vi "display_michelle_PTK_visjitter_stopadded_RandCont_PsuedoCO_TSLog.vi"() -> ()   [LabVIEW 2019]
uses:
  <vilib>/Analysis/Matrix/Datatypes/RealMatrix.ctl
  <vilib>/Utility/file.llb/Write Delimited Spreadsheet (DBL).vi
  <vilib>/Analysis/Matrix/NI_Matrix.lvlib
panel:
  out "lambda":dbl
  out "maxITI":dbl
  out "minITI":dbl
  out "goEXP":dbl
  out "meanITI":dbl
  out "Lag1":dbl
  out "TSLog":dbl[][](array[numeric])
  out "TSLog2":dbl[][](array[numeric])
  out "Initialtime":dbl
  out "Time Stamp":timestamp format="%<%H:%M:%S%4u>T"
  out "TSLog1":dbl[][](array[numeric])
  out "ArrayTemp3":T1
  out "StimID2":dbl
  out "Contrast":dbl
  out "TimeOutCounter":i32
  out "ElapsedTime_M":dbl
  out "Base_Contrast":dbl
  out "CurrentTrial":u32=1
  out "Jitter":dbl
  out "BaseITI":dbl
  out "VisStimDuration":dbl
  in  "Stop":bool
  out "Num trials":u32=204
  out "ISI Time":dbl
  out "Stim TS":dbl
  out "Output":dbl[][](array[numeric])
  out "Output frame":T1
  out "Array temp1":T1
  out "Elapsed Time":dbl
  out "Display":bool=TRUE
  out "Trial":u32=1
  out "reward":dbl[](array[numeric])
  out "stim_id":dbl[](array[numeric])
  out "stim_loaded":dbl
  out "Timings":dbl[](array[numeric])
  out "Stimuli Loaded?":bool
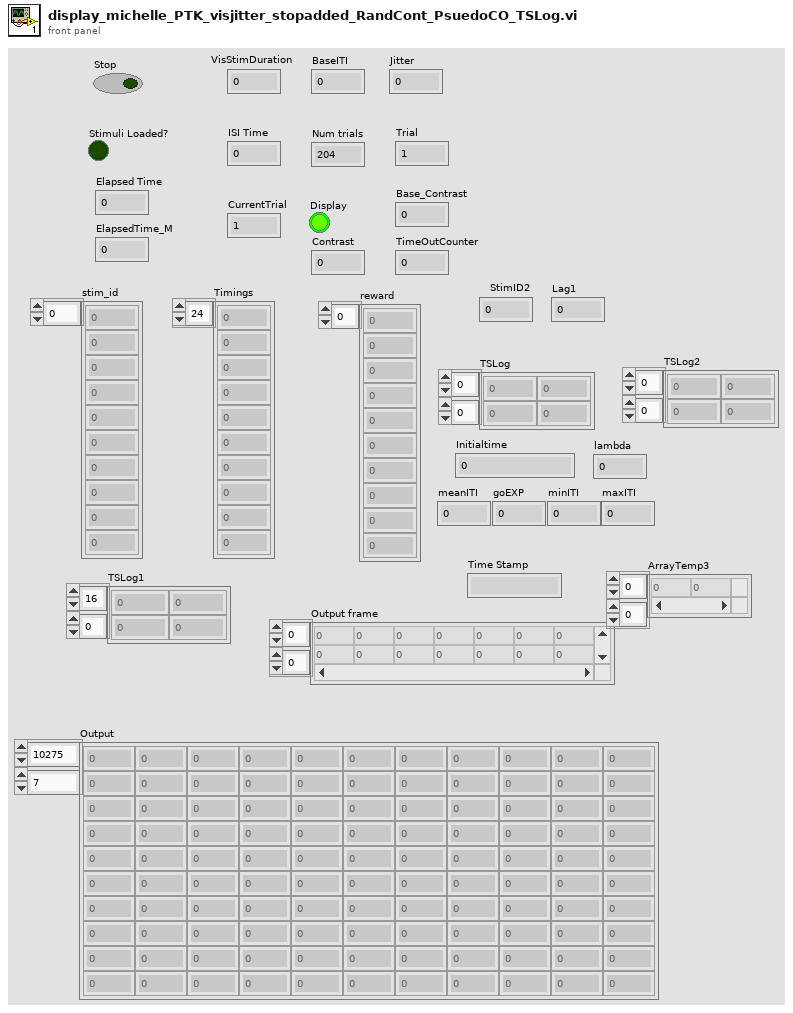
[diagram p1: front panel]
types:
  T1 = typedef "NI_Matrix.lvlib/RealMatrix.ctl" = dbl[][]
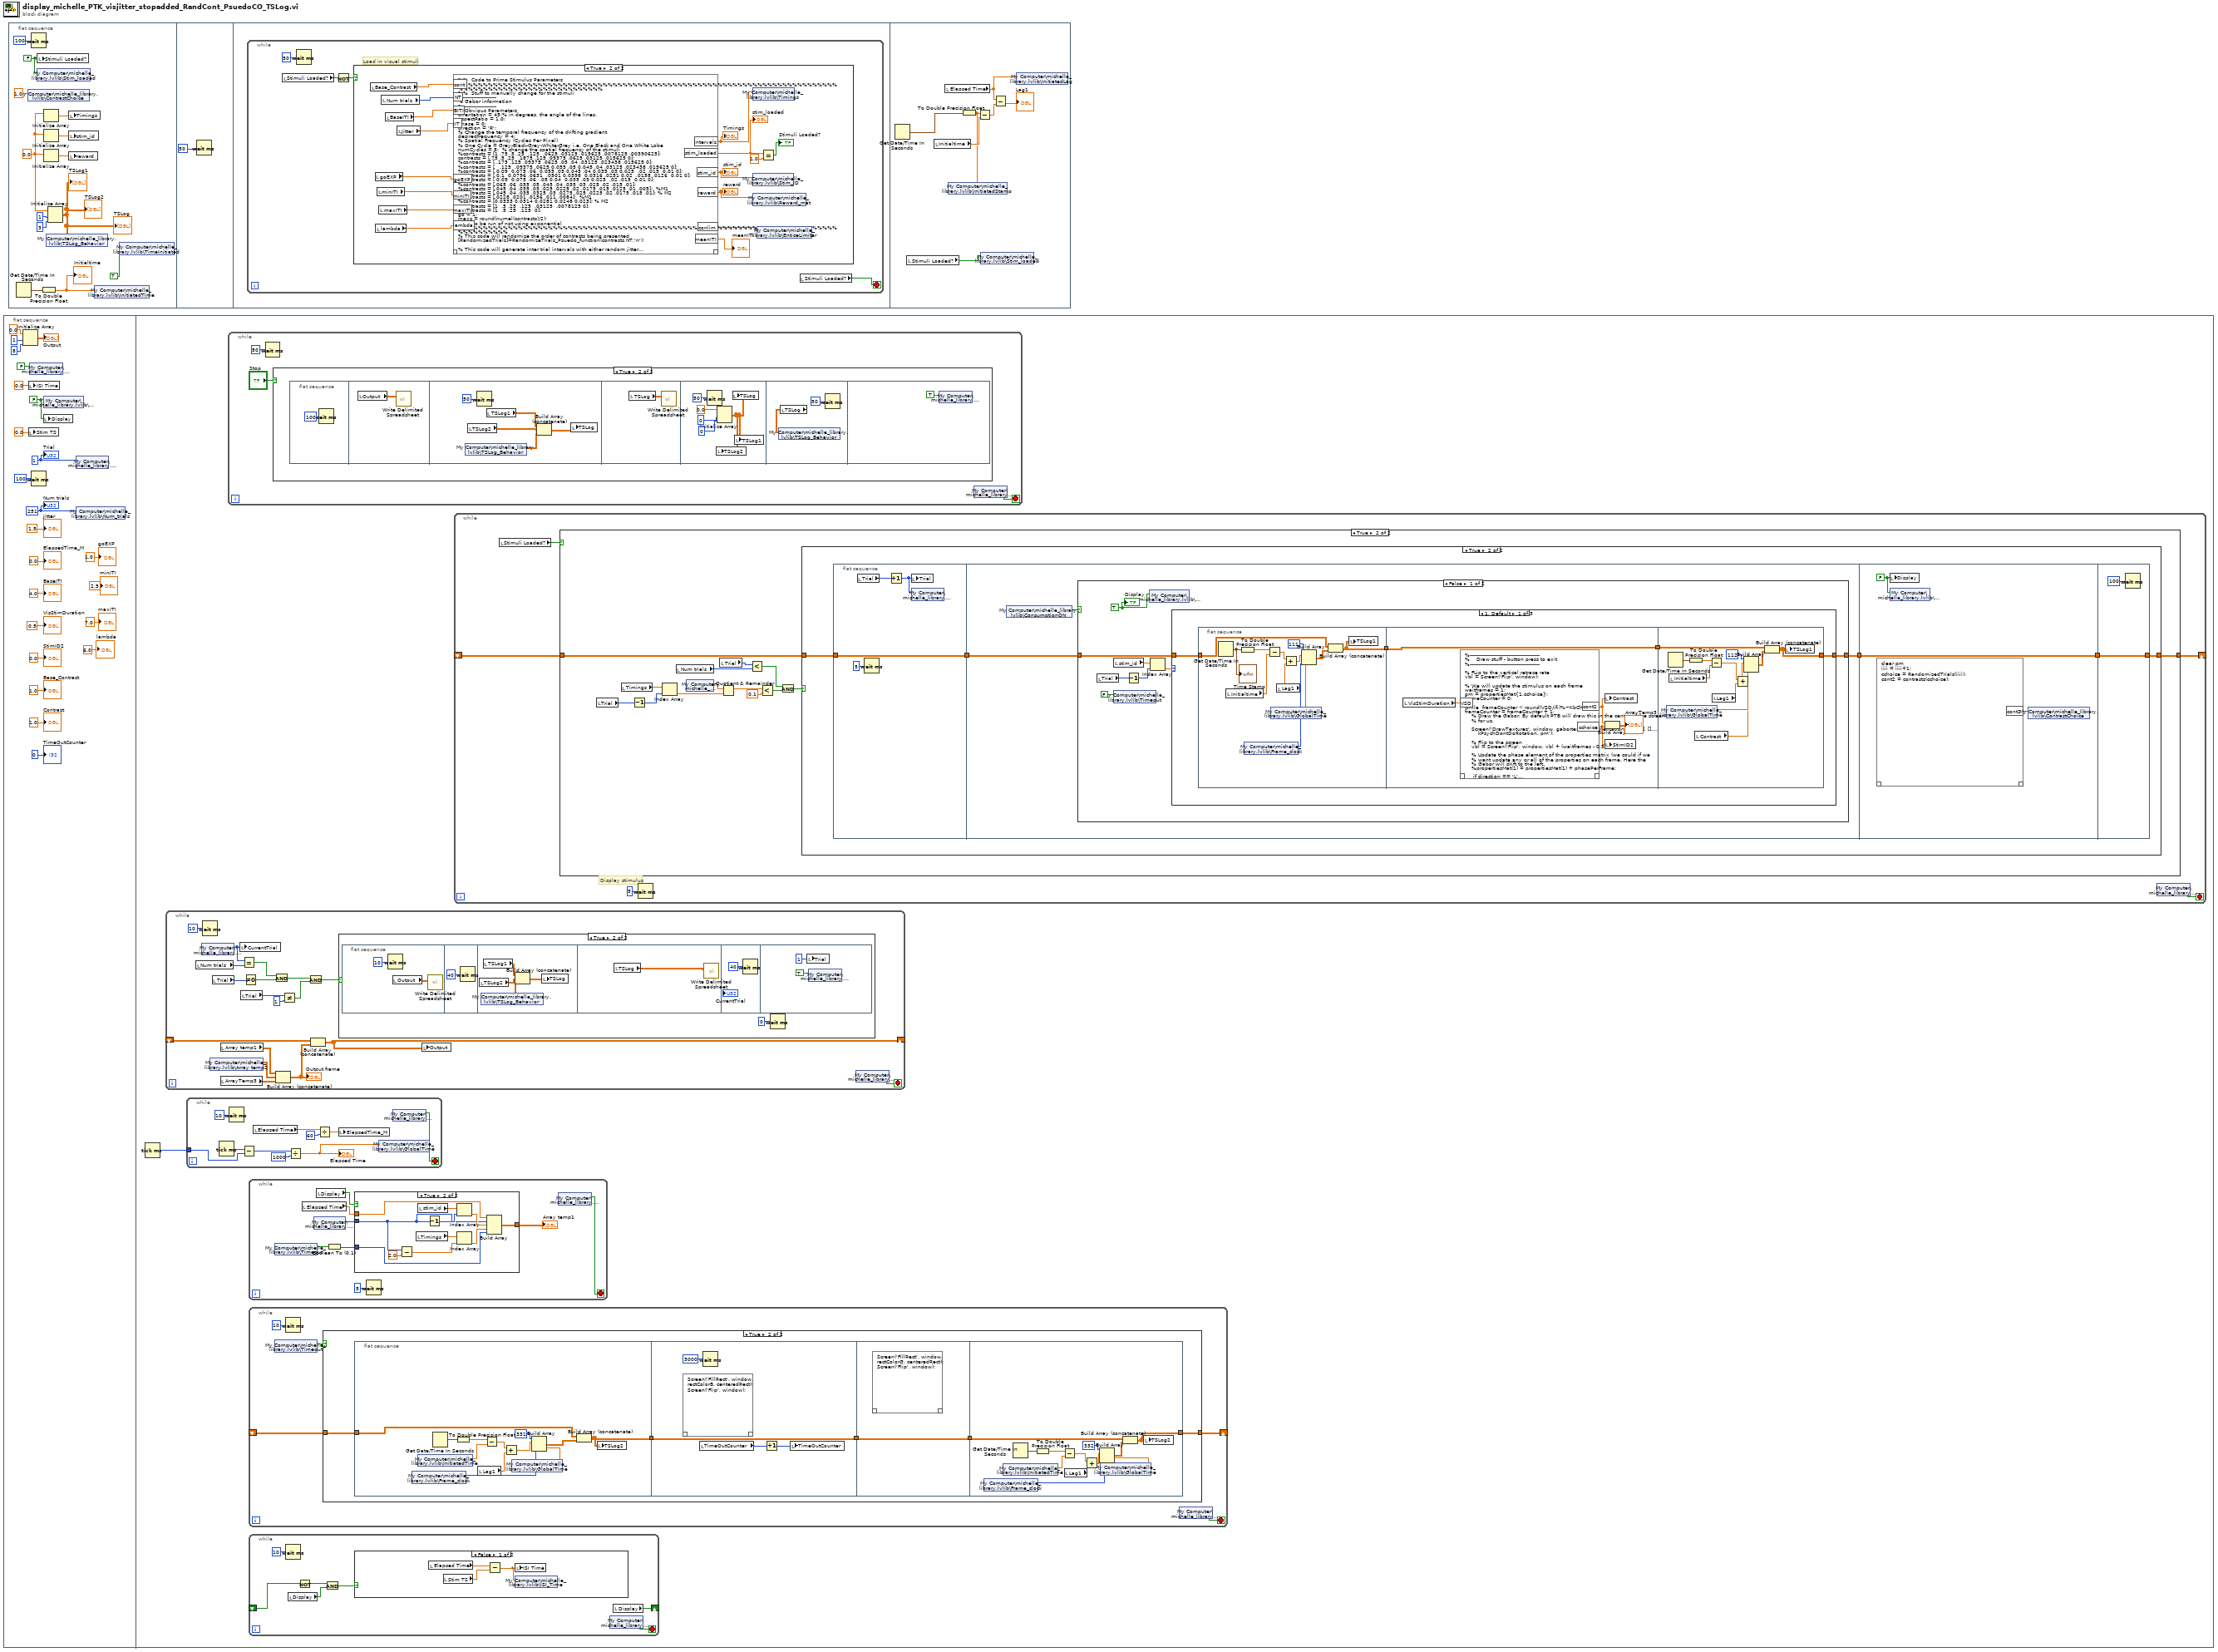
[diagram p0: block diagram]
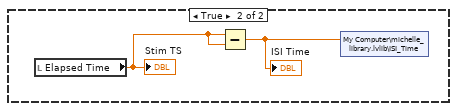
[diagram p5: hidden frame]
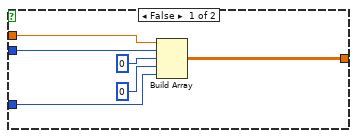
[diagram p6: hidden frame]
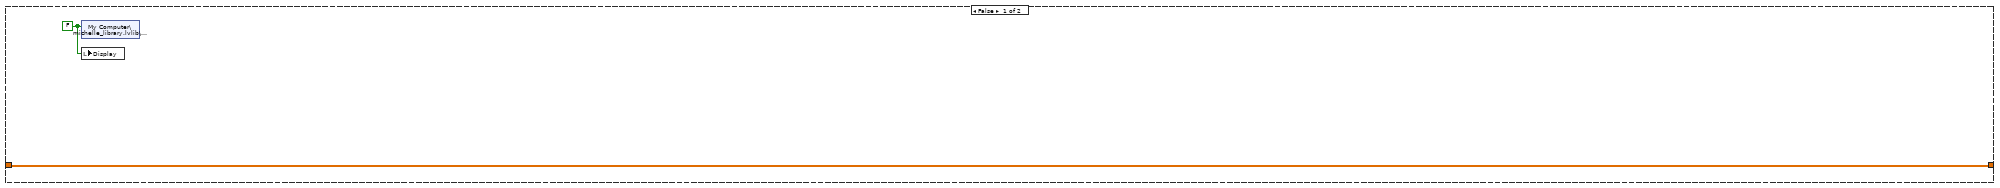
[diagram p9: hidden frame]
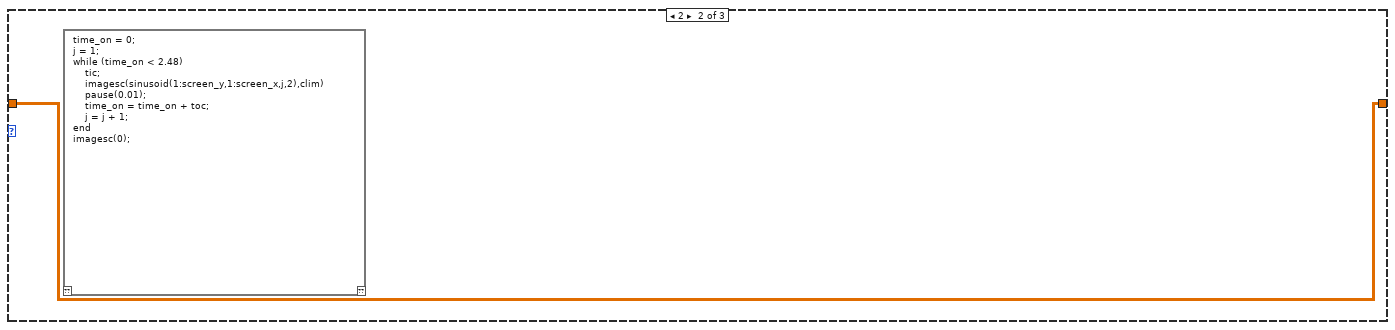
[diagram p10: hidden frame]
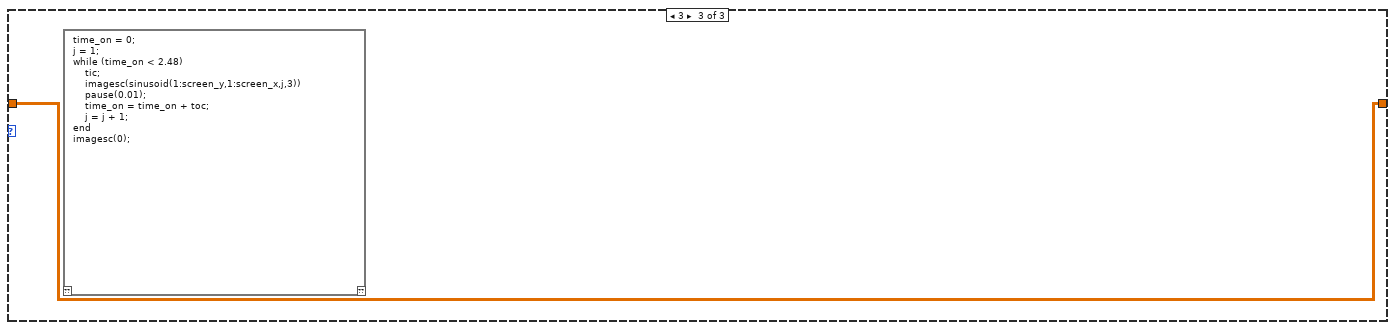
[diagram p11: hidden frame]
diagram:
  n1 = flat-sequence {
    frame #0 {
      w15 = u32 251
      w21 = FALSE ("Display")
      w23 = u32 1 ("Trial")
      n2 = Initialize Array(0.0 ("element"), 1 ("dimension size"), 8 ("dimension size")) -> (→"Output":dbl[][])
      n3 = local write "ISI Time"(0.0 ("ISI Time")) -> ()
      n4 = local write "Stim TS"(0.0 ("Stim TS")) -> ()
      n5 = shared-variable "My Computer\\michelle_library.lvlib\\Stop"(FALSE ("Stop")) -> ()  [unwired: 1 in, 1 out]
      n6 = Wait (ms)(milliseconds to wait=u32 100) -> ()  [unwired: 1 out]
      n7 = shared-variable "My Computer\\michelle_library.lvlib\\Display"(w21) -> ()  [unwired: 1 in, 1 out]
      n8 = local write "Display"(w21) -> ()
      n9 = shared-variable "My Computer\\michelle_library.lvlib\\Trial"(w23) -> ()  [unwired: 1 in, 1 out]
      n10 = shared-variable "My Computer\\michelle_library.lvlib\\Num_trials"(w15) -> ()  [unwired: 1 in, 1 out]
      "Trial" <- w23
      "Num trials" <- w15
      "VisStimDuration" <- 0.5
      "BaseITI" <- 4.0
      "Jitter" <- 1.5
      "Base_Contrast" <- 1.0
      "ElapsedTime_M" <- 0.0
      "TimeOutCounter" <- 0
      "Contrast" <- 1.0
      "StimID2" <- 0.0
      "goEXP" <- 1.0
      "minITI" <- 2.5
      "maxITI" <- 7.0
      "lambda" <- 6.0
    }
    frame #1 {
      n11 = Tick Count (ms)() -> (millisecond timer value=w24:u32)
      n12 = while {
        shift-right: [w145] -> _
        shift-left: _ -> [w146]
        stop <- w148 stop-if-true
        n13 = local read "Num trials"() -> (w141:u32)
        n14 = shared-variable "My Computer\\michelle_library.lvlib\\Trial"() -> (w132:u32)  [unwired: 1 in, 1 out]
        n15 = Wait (ms)(milliseconds to wait=u32 10) -> ()  [unwired: 1 out]
        n16 = shared-variable "My Computer\\michelle_library.lvlib\\Array temp2"() -> (w143:dbl[][])  [unwired: 1 in, 1 out]
        n17 = local read "Trial"() -> (w139:u32)
        n18 = local read "Array temp1"() -> (w144:T1)
        n19 = local read "ArrayTemp3"() -> (w131:T1)
        n20 = local write "CurrentTrial"(w132) -> ()
        n21 = local read "Trial"() -> (w138:u32)
        n22 = Equal?(x=w132, y=w141) -> (x = y?=w140:bool)
        n23 = Not Equal To 0?(x=w139) -> (x != 0?=w135:bool)
        n24 = And(x=w140, y=w135) -> (x .and. y?=w133:bool)
        n25 = Build Array (concatenate)(w144, w143, w131) -> (w142:T1)
        "Output frame" <- w142
        n26 = Not Equal?(x=w138, y=1) -> (x != y?=w137:bool)
        n27 = And(x=w133, y=w137) -> (x .and. y?=w134:bool)
        n28 = Build Array (concatenate) ("Build Matrix")(w146, w142) -> (w145:T1)
        n29 = case shown="True" w134 {
          frame False {
          }
          frame True {
            n30 = flat-sequence {
              frame #0 {
                n31 = Wait (ms)(milliseconds to wait=u32 10) -> ()  [unwired: 1 out]
                n32 = local read "Output"() -> (w151:dbl[][])
                n33 = call-poly <vilib>:"Write Delimited Spreadsheet.vi"("2D data"=w151) -> ()  [unwired: 13 in, 2 out]
              }
              frame #1 {
                n34 = Wait (ms)(milliseconds to wait=u32 40) -> ()  [unwired: 1 out]
              }
              frame #2 {
                n35 = local read "TSLog2"() -> (w156:dbl[][])
                n36 = shared-variable "My Computer\\michelle_library.lvlib\\TSLog_Behavior"() -> (w154:dbl[][])  [unwired: 1 in, 1 out]
                n37 = local read "TSLog1"() -> (w155:dbl[][])
                n38 = Build Array (concatenate) ("Build Matrix")(w155, w156, w154) -> (w153:T1)
                n39 = local write "TSLog"(w153) -> ()
              }
              frame #3 {
                n40 = local read "TSLog"() -> (w157:dbl[][])
                n41 = call-poly <vilib>:"Write Delimited Spreadsheet.vi"("2D data"=w157) -> ()  [unwired: 13 in, 2 out]
              }
              frame #4 {
                n42 = Wait (ms)(milliseconds to wait=u32 40) -> ()  [unwired: 1 out]
              }
              frame #5 {
                n43 = local write "Trial"(1) -> ()
                n44 = shared-variable "My Computer\\michelle_library.lvlib\\Stop"(TRUE) -> ()  [unwired: 1 in, 1 out]
              }
            }
            n45 = Wait (ms)(milliseconds to wait=0) -> ()  [unwired: 1 out]
          }
        }
        n46 = local write "Output"(w145) -> ()
        n47 = shared-variable "My Computer\\michelle_library.lvlib\\Stop"() -> (w148:bool)  [unwired: 1 in, 1 out]
      }
      n48 = while {
        tunnel: w24 -> [w128]
        stop <- w125 stop-if-true
        n49 = Tick Count (ms)() -> (millisecond timer value=w129:u32)
        n50 = Wait (ms)(milliseconds to wait=u32 10) -> ()  [unwired: 1 out]
        n51 = Subtract(x=w129, y=w128) -> (x-y=w126:u32)
        n52 = local read "Elapsed Time"() -> (w123:dbl)
        n53 = Divide(x=w126, y=u32 1000) -> (x/y=w121:dbl)
        "Elapsed Time" <- w121
        n54 = Divide(x=w123, y=60) -> (x/y=w122:dbl)
        n55 = local write "ElapsedTime_M"(w122) -> ()
        n56 = shared-variable "My Computer\\michelle_library.lvlib\\GlobalTime"(w121) -> ()  [unwired: 1 in, 1 out]
        n57 = shared-variable "My Computer\\michelle_library.lvlib\\Stop"() -> (w125:bool)  [unwired: 1 in, 1 out]
      }
      n58 = while {
        stop <- w27 stop-if-true
        n59 = Wait (ms)(milliseconds to wait=50) -> ()  [unwired: 1 out]
        n60 = case shown="True" "Stop" {
          frame False {
          }
          frame True {
            n61 = flat-sequence {
              frame #0 {
                n62 = Wait (ms)(milliseconds to wait=100) -> ()  [unwired: 1 out]
              }
              frame #1 {
                n63 = local read "Output"() -> (w29:dbl[][])
                n64 = call-poly <vilib>:"Write Delimited Spreadsheet.vi"("2D data"=w29) -> ()  [unwired: 13 in, 2 out]
              }
              frame #2 {
                n65 = shared-variable "My Computer\\michelle_library.lvlib\\TSLog_Behavior"() -> (w30:dbl[][])  [unwired: 1 in, 1 out]
                n66 = local read "TSLog2"() -> (w33:dbl[][])
                n67 = Wait (ms)(milliseconds to wait=50) -> ()  [unwired: 1 out]
                n68 = local read "TSLog1"() -> (w32:dbl[][])
                n69 = Build Array (concatenate) ("Build Matrix")(w32, w33, w30) -> (w31:T1)
                n70 = local write "TSLog"(w31) -> ()
              }
              frame #3 {
                n71 = local read "TSLog"() -> (w35:dbl[][])
                n72 = call-poly <vilib>:"Write Delimited Spreadsheet.vi"("2D data"=w35) -> ()  [unwired: 13 in, 2 out]
              }
              frame #4 {
                n73 = Wait (ms)(milliseconds to wait=50) -> ()  [unwired: 1 out]
                n74 = Initialize Array(0.0, 0, 0) -> (w37:dbl[][])
                n75 = local write "TSLog2"(w37) -> ()
                n76 = local write "TSLog"(w37) -> ()
                n77 = local write "TSLog1"(w37) -> ()
              }
              frame #5 {
                n78 = local read "TSLog"() -> (w42:dbl[][])
                n79 = shared-variable "My Computer\\michelle_library.lvlib\\TSLog_Behavior"(w42) -> ()  [unwired: 1 in, 1 out]
                n80 = Wait (ms)(milliseconds to wait=50) -> ()  [unwired: 1 out]
              }
              frame #6 {
                n81 = shared-variable "My Computer\\michelle_library.lvlib\\Stop"(TRUE) -> ()  [unwired: 1 in, 1 out]
              }
            }
          }
        }
        n82 = shared-variable "My Computer\\michelle_library.lvlib\\Stop"() -> (w27:bool)  [unwired: 1 in, 1 out]
      }
      n83 = while {
        stop <- w98 stop-if-true
        n84 = shared-variable "My Computer\\michelle_library.lvlib\\Timeout"() -> (w96:bool)  [unwired: 1 in, 1 out]
        n85 = local read "Elapsed Time"() -> (w102:dbl)
        n86 = shared-variable "My Computer\\michelle_library.lvlib\\Trial"() -> (w100:u32)  [unwired: 1 in, 1 out]
        n87 = local read "Display"() -> (w99:bool)
        n88 = Boolean To (0,1)(Boolean=w96) -> (0, 1=w97:i16)
        n89 = case shown="True" w99 {
          tunnel: w100 -> [w108 w111]
          tunnel: w102 -> [w109 w118]
          tunnel: [w107 w119] -> w101
          tunnel: w97 -> [w104 w113]
          frame False {
            n90 = Build Array(w109, w108, u32 0 ("milliseconds to wait"), 0, w104) -> (w107:T1)
          }
          frame True {
            n91 = Subtract(x=w111, y=2.0) -> (x-y=w110:dbl)
            n92 = local read "Timings"() -> (w116:dbl[])
            n93 = local read "stim_id"() -> (w120:dbl[])
            n94 = Decrement(x=w111) -> (x-1=w115:u32)
            n95 = Index Array(array=w120, index=w115) -> (element=w117:dbl)
            n96 = Index Array(array=w116, index=w110) -> (element=w114:dbl)
            n97 = Build Array(w118, w111, w117, w114, w113) -> (w119:T1)
          }
        }
        "Array temp1" <- w101
        n98 = Wait (ms)(milliseconds to wait=u32 5) -> ()  [unwired: 1 out]
        n99 = shared-variable "My Computer\\michelle_library.lvlib\\Stop"() -> (w98:bool)  [unwired: 1 in, 1 out]
      }
      n100 = while {
        shift-right: [w44] -> _
        shift-left: _ -> [w45]
        stop <- w48 stop-if-true
        n101 = shared-variable "My Computer\\michelle_library.lvlib\\Timeout"() -> (w46:bool)  [unwired: 1 in, 1 out]
        n102 = Wait (ms)(milliseconds to wait=u32 10) -> ()  [unwired: 1 out]
        n103 = case shown="True" w46 {
          tunnel: w45 -> [w49 w54]
          tunnel: [w49 w53] -> w44
          frame False {
          }
          frame True {
            n104 = flat-sequence {
              tunnel: w54 -> [w61]
              tunnel: [w60] -> w51
              tunnel: [w67] -> w52
              tunnel: w51 -> [w67]
              tunnel: w52 -> [w71]
              tunnel: [w71] -> w50
              tunnel: [w77] -> w53
              tunnel: w50 -> [w78]
              frame #0 {
                n105 = shared-variable "My Computer\\michelle_library.lvlib\\Frame_clock"() -> (w55:u32)  [unwired: 1 in, 1 out]
                n106 = shared-variable "My Computer\\michelle_library.lvlib\\InitiatedTime"() -> (w64:dbl)  [unwired: 1 in, 1 out]
                n107 = Get Date/Time In Seconds() -> (seconds since 1Jan1904=w66:timestamp)
                n108 = To Double Precision Float(number=w66) -> (double precision float=w65:dbl)
                n109 = local read "Lag1"() -> (w57:dbl)
                n110 = Subtract(x=w65, y=w64) -> (x-y=w58:dbl)
                n111 = Add(x=w58, y=w57) -> (x+y=w59:dbl)
                n112 = shared-variable "My Computer\\michelle_library.lvlib\\GlobalTime"() -> (w56:dbl)  [unwired: 1 in, 1 out]
                n113 = Build Array(331, w59, w56, w55) -> (w63:T1)
                n114 = Build Array (concatenate) ("Build Matrix")(w61, w63) -> (w60:T1)
                n115 = local write "TSLog2"(w60) -> ()
              }
              frame #1 {
                n116 = script code="Screen('FillRect', window, rectColorB, centeredRect);\nScreen('Flip', window);"() -> ()  [unwired: 1 in, 1 out]
                n117 = local read "TimeOutCounter"() -> (w69:i32)
                n118 = Wait (ms)(milliseconds to wait=u32 3000) -> ()  [unwired: 1 out]
                n119 = Increment(x=w69) -> (x+1=w68:i32)
                n120 = local write "TimeOutCounter"(w68) -> ()
              }
              frame #2 {
                n121 = script code="Screen('FillRect', window, rectColorG, centeredRect);\nScreen('Flip', window);"() -> ()  [unwired: 1 in, 1 out]
              }
              frame #3 {
                n122 = shared-variable "My Computer\\michelle_library.lvlib\\Frame_clock"() -> (w72:u32)  [unwired: 1 in, 1 out]
                n123 = shared-variable "My Computer\\michelle_library.lvlib\\InitiatedTime"() -> (w83:dbl)  [unwired: 1 in, 1 out]
                n124 = Get Date/Time In Seconds() -> (seconds since 1Jan1904=w81:timestamp)
                n125 = To Double Precision Float(number=w81) -> (double precision float=w82:dbl)
                n126 = Subtract(x=w82, y=w83) -> (x-y=w75:dbl)
                n127 = local read "Lag1"() -> (w74:dbl)
                n128 = Add(x=w75, y=w74) -> (x+y=w76:dbl)
                n129 = shared-variable "My Computer\\michelle_library.lvlib\\GlobalTime"() -> (w73:dbl)  [unwired: 1 in, 1 out]
                n130 = Build Array(332, w76, w73, w72) -> (w79:T1)
                n131 = Build Array (concatenate) ("Build Matrix")(w78, w79) -> (w77:T1)
                n132 = local write "TSLog2"(w77) -> ()
              }
            }
          }
        }
        n133 = shared-variable "My Computer\\michelle_library.lvlib\\Stop"() -> (w48:bool)  [unwired: 1 in, 1 out]
      }
      n134 = while {
        shift-right: [w88] -> _
        shift-left: _ -> [w87]
        stop <- w90 stop-if-true
        n135 = Wait (ms)(milliseconds to wait=u32 10) -> ()  [unwired: 1 out]
        n136 = local read "Display"() -> (w85:bool)
        n137 = Not(x=w87) -> (.not. x?=w86:bool)
        n138 = And(x=w86, y=w85) -> (x .and. y?=w84:bool)
        n139 = case shown="False" w84 {
          frame False {
            n140 = local read "Elapsed Time"() -> (w91:dbl)
            n141 = local read "Stim TS"() -> (w93:dbl)
            n142 = Subtract(x=w91, y=w93) -> (x-y=w92:dbl)
            n143 = local write "ISI Time"(w92) -> ()
            n144 = shared-variable "My Computer\\michelle_library.lvlib\\ISI_Time"(w92) -> ()  [unwired: 1 in, 1 out]
          }
          frame True {
            n145 = local read "Elapsed Time"() -> (w94:dbl)
            "Stim TS" <- w94
            n146 = Subtract(x=w94, y=w94) -> (x-y=w95:dbl)
            "ISI Time" <- w95
            n147 = shared-variable "My Computer\\michelle_library.lvlib\\ISI_Time"(w95) -> ()  [unwired: 1 in, 1 out]
          }
        }
        n148 = shared-variable "My Computer\\michelle_library.lvlib\\Stop"() -> (w90:bool)  [unwired: 1 in, 1 out]
        n149 = local read "Display"() -> (w88:bool)
      }
      n150 = while {
        shift-right: [w161] -> _
        shift-left: _ -> [w162]
        stop <- w164 stop-if-true
        # "Display stimulus"
        n151 = local read "Stimuli Loaded?"() -> (w163:bool)
        n152 = case shown="True" w163 {
          tunnel: w162 -> [w166 w168]
          tunnel: [w166 w167] -> w161
          frame False {
          }
          frame True {
            n153 = local read "Trial"() -> (w169:u32)
            n154 = local read "Timings"() -> (w178:dbl[])
            n155 = Decrement(x=w169) -> (x-1=w170:u32)
            n156 = Index Array(array=w178, index=w170) -> (element=w177:dbl)
            n157 = local read "Num trials"() -> (w173:u32)
            n158 = shared-variable "My Computer\\michelle_library.lvlib\\ISI"() -> (w172:dbl)  [unwired: 1 in, 1 out]
            n159 = local read "Trial"() -> (w176:u32)
            n160 = Quotient & Remainder(x=w172, y=w177) -> (x-y*floor(x/y)=w180:dbl)  [unwired: 1 out]
            n161 = Less?(x=w176, y=w173) -> (x < y?=w175:bool)
            n162 = Less?(x=w180, y=0.1) -> (x < y?=w174:bool)
            n163 = And(x=w175, y=w174) -> (x .and. y?=w171:bool)
            n164 = case shown="True" w171 {
              tunnel: w168 -> [w181 w186]
              tunnel: [w181 w185] -> w167
              frame False {
                w182 = FALSE ("Display")
                n165 = shared-variable "My Computer\\michelle_library.lvlib\\Display"(w182) -> ()  [unwired: 1 in, 1 out]
                n166 = local write "Display"(w182) -> ()
              }
              frame True {
                n167 = flat-sequence {
                  tunnel: [w188] -> w187
                  tunnel: w186 -> [w188]
                  tunnel: w187 -> [w193]
                  tunnel: [w192] -> w183
                  tunnel: [w239] -> w184
                  tunnel: w183 -> [w239]
                  tunnel: [w242] -> w185
                  tunnel: w184 -> [w242]
                  frame #0 {
                    n168 = local read "Trial"() -> (w191:u32)
                    n169 = Wait (ms)(milliseconds to wait=u32 5) -> ()  [unwired: 1 out]
                    n170 = Increment(x=w191) -> (x+1=w190:u32)
                    n171 = local write "Trial"(w190) -> ()
                    n172 = shared-variable "My Computer\\michelle_library.lvlib\\Trial"(w190) -> ()  [unwired: 1 in, 1 out]
                  }
                  frame #1 {
                    n173 = shared-variable "My Computer\\michelle_library.lvlib\\ConsumptionON"() -> (w194:bool)  [unwired: 1 in, 1 out]
                    n174 = case shown="False" w194 {
                      tunnel: w193 -> [w196 w238]
                      tunnel: [w195 w238] -> w192
                      frame False {
                        w197 = TRUE ("Boolean")
                        n175 = local read "Trial"() -> (w200:u32)
                        n176 = shared-variable "My Computer\\michelle_library.lvlib\\Timeout"(FALSE) -> ()  [unwired: 1 in, 1 out]
                        n177 = local read "stim_id"() -> (w202:dbl[])
                        n178 = Decrement(x=w200) -> (x-1=w199:u32)
                        n179 = shared-variable "My Computer\\michelle_library.lvlib\\Display"(w197) -> ()  [unwired: 1 in, 1 out]
                        n180 = Index Array(array=w202, index=w199) -> (element=w201:dbl)
                        n181 = case shown="1, Default" w201 {
                          tunnel: w196 -> [w206 w236 w237]
                          tunnel: [w205 w236 w237] -> w195
                          frame 1, Default {
                            n182 = flat-sequence {
                              tunnel: w206 -> [w217]
                              tunnel: [w216] -> w204
                              tunnel: w204 -> [w219]
                              tunnel: [w219] -> w203
                              tunnel: [w234] -> w205
                              tunnel: w203 -> [w233]
                              frame #0 {
                                n183 = Get Date/Time In Seconds() -> (seconds since 1Jan1904=w214:timestamp)
                                "Time Stamp" <- w214
                                n184 = local read "Initialtime"() -> (w212:dbl)
                                n185 = To Double Precision Float(number=w214) -> (double precision float=w213:dbl)
                                n186 = shared-variable "My Computer\\michelle_library.lvlib\\Frame_clock"() -> (w207:u32)  [unwired: 1 in, 1 out]
                                n187 = Subtract(x=w213, y=w212) -> (x-y=w210:dbl)
                                n188 = shared-variable "My Computer\\michelle_library.lvlib\\GlobalTime"() -> (w208:dbl)  [unwired: 1 in, 1 out]
                                n189 = local read "Lag1"() -> (w211:dbl)
                                n190 = Add(x=w210, y=w211) -> (x+y=w209:dbl)
                                n191 = Build Array(111, w209, w208, w207) -> (w215:T1)
                                n192 = Build Array (concatenate) ("Build Matrix")(w217, w215) -> (w216:T1)
                                n193 = local write "TSLog1"(w216) -> ()
                              }
                              frame #1 {
                                n194 = local read "VisStimDuration"() -> (w221:dbl)
                                n195 = script code="%------------------------------------------\n%    Draw stuff - button press to exit\n%------------------------------------------\n\n% FLip to the vertical retrace rate\nvbl = Screen('Flip', window);\n\n% We will update the stimulus on each frame\nwaitframes = 1;\npm = propertiesMat{1,cchoice};\nframeCounter = 0;\ntic\nwhile  frameCounter < round(VSD/ifi)%~KbCheck\nframeCounter = frameCounter + 1;\n    % Draw the Gabor. By default PTB will draw this in the center of the screen\n    % for us.\n   \n    Screen('DrawTextures', window, gabortex, [], [], orientation, [], [], [], [],...\n        kPsychDontDoRotation, pm');\n\n    % Flip to the screen\n    vbl = Screen('Flip', window, vbl + (waitframes - 0.5) * ifi);\n\n    % Update the phase element of the properties matrix (we could if we\n    % want update any or all of the properties on each frame. Here the\n    % Gabor will drift to the left.\n    %propertiesMat(1) = propertiesMat(1) + phasePerFrame;\n \n     if direction == 'L'\n          pm(1) = pm(1) + phasePerFrame;\n     elseif direction =='R'\n          pm(1) = pm(1) - phasePerFrame;\n     end\n\nend\nTime(N) = toc;\nvbl = Screen('Flip', window);"("VSD"=w221) -> ("cont2"=w223:dbl, "cchoice"=w222:dbl)  [unwired: 1 in, 1 out]
                                n196 = local write "Contrast"(w223) -> ()
                                n197 = Build Array(w223, w222) -> (→"ArrayTemp3":T1)
                                n198 = local write "StimID2"(w222) -> ()
                              }
                              frame #2 {
                                n199 = shared-variable "My Computer\\michelle_library.lvlib\\GlobalTime"() -> (w225:dbl)  [unwired: 1 in, 1 out]
                                n200 = Get Date/Time In Seconds() -> (seconds since 1Jan1904=w231:timestamp)
                                n201 = local read "Initialtime"() -> (w230:dbl)
                                n202 = To Double Precision Float(number=w231) -> (double precision float=w229:dbl)
                                n203 = local read "Contrast"() -> (w224:dbl)
                                n204 = Subtract(x=w229, y=w230) -> (x-y=w228:dbl)
                                n205 = local read "Lag1"() -> (w226:dbl)
                                n206 = Add(x=w228, y=w226) -> (x+y=w227:dbl)
                                n207 = Build Array(112, w227, w225, w224) -> (w235:T1)
                                n208 = Build Array (concatenate) ("Build Matrix")(w233, w235) -> (w234:T1)
                                n209 = local write "TSLog1"(w234) -> ()
                              }
                            }
                          }
                          frame 2 {
                            n210 = script code="time_on = 0;\nj = 1;\nwhile (time_on < 2.48)\n    tic;\n    imagesc(sinusoid(1:screen_y,1:screen_x,j,2),clim)\n    pause(0.01);\n    time_on = time_on + toc;\n    j = j + 1;\nend\nimagesc(0);"() -> ()  [unwired: 1 in, 1 out]
                          }
                          frame 3 {
                            n211 = script code="time_on = 0;\nj = 1;\nwhile (time_on < 2.48)\n    tic;\n    imagesc(sinusoid(1:screen_y,1:screen_x,j,3))\n    pause(0.01);\n    time_on = time_on + toc;\n    j = j + 1;\nend\nimagesc(0);"() -> ()  [unwired: 1 in, 1 out]
                          }
                        }
                        "Display" <- w197
                      }
                      frame True {
                      }
                    }
                  }
                  frame #2 {
                    w241 = FALSE ("Display")
                    n212 = script code="clear pm\niiii = iiii+1;\ncchoice = RandomizedTrials(iiii);\ncont2 = contrasts(cchoice);"() -> ("cont2"=w240:dbl)  [unwired: 1 in, 1 out]
                    n213 = local write "Display"(w241) -> ()
                    n214 = shared-variable "My Computer\\michelle_library.lvlib\\Display"(w241) -> ()  [unwired: 1 in, 1 out]
                    n215 = shared-variable "My Computer\\michelle_library.lvlib\\ContrastChoice"(w240) -> ()  [unwired: 1 in, 1 out]
                  }
                  frame #3 {
                    n216 = Wait (ms)(milliseconds to wait=u32 100) -> ()  [unwired: 1 out]
                  }
                }
              }
            }
          }
        }
        n217 = Wait (ms)(milliseconds to wait=u32 5) -> ()  [unwired: 1 out]
        n218 = shared-variable "My Computer\\michelle_library.lvlib\\Stop"() -> (w164:bool)  [unwired: 1 in, 1 out]
      }
    }
  }
  n219 = flat-sequence {
    frame #0 {
      w250 = 0.0 ("element")
      w252 = FALSE ("Stimuli Loaded?")
      n220 = Get Date/Time In Seconds() -> (seconds since 1Jan1904=w247:timestamp)
      n221 = shared-variable "My Computer\\michelle_library.lvlib\\ContrastChoice"(1.0) -> ()  [unwired: 1 in, 1 out]
      n222 = Wait (ms)(milliseconds to wait=u32 100) -> ()  [unwired: 1 out]
      n223 = local write "Stimuli Loaded?"(w252) -> ()
      n224 = shared-variable "My Computer\\michelle_library.lvlib\\Stim_loaded"(w252) -> ()  [unwired: 1 in, 1 out]
      n225 = To Double Precision Float(number=w247) -> (double precision float=w246:dbl)
      "Initialtime" <- w246
      n226 = Initialize Array(w250) -> (w255:dbl[])  [unwired: 1 in]
      n227 = Initialize Array(w250) -> (w254:dbl[])  [unwired: 1 in]
      n228 = Initialize Array(w250) -> (w253:dbl[])  [unwired: 1 in]
      n229 = Initialize Array(w250, 1, 3) -> (w244:dbl[][])
      "TSLog1" <- w244
      "TSLog2" <- w244
      "TSLog" <- w244
      n230 = shared-variable "My Computer\\michelle_library.lvlib\\TSLog_Behavior"(w244) -> ()  [unwired: 1 in, 1 out]
      n231 = local write "Timings"(w255) -> ()
      n232 = local write "stim_id"(w254) -> ()
      n233 = local write "reward"(w253) -> ()
      n234 = shared-variable "My Computer\\michelle_library.lvlib\\InitiatedTime"(w246) -> ()  [unwired: 1 in, 1 out]
      n235 = shared-variable "My Computer\\michelle_library.lvlib\\TimeInitiated"(TRUE) -> ()  [unwired: 1 in, 1 out]
    }
    frame #1 {
      n236 = Wait (ms)(milliseconds to wait=u32 50) -> ()  [unwired: 1 out]
    }
    frame #2 {
      n237 = while {
        stop <- w258 stop-if-true
        # "Load in visual stimuli"
        n238 = local read "Stimuli Loaded?"() -> (w260:bool)
        n239 = Wait (ms)(milliseconds to wait=u32 50) -> ()  [unwired: 1 out]
        n240 = Not(x=w260) -> (.not. x?=w259:bool)
        n241 = case shown="True" w259 {
          frame False {
          }
          frame True {
            n242 = local read "Base_Contrast"() -> (w269:dbl)
            n243 = local read "goEXP"() -> (w265:dbl)
            n244 = local read "lambda"() -> (w262:dbl)
            n245 = local read "minITI"() -> (w264:dbl)
            n246 = local read "maxITI"() -> (w263:dbl)
            n247 = local read "Num trials"() -> (w272:u32)
            n248 = local read "BaseITI"() -> (w271:dbl)
            n249 = local read "Jitter"() -> (w270:dbl)
            n250 = script code="%%  Code to Prime Stimulus Parameters\n%%%%%%%%%%%%%%%%%%%%%%%%%%%%%%%%%%%%%%%%%%%%%%%%%%%%%%%%%%%%%%%%%%%%%%%%%%%%%%%%%%%%%%%%%%%%%%%%%%%%%%%%%\n%%  Stuff to manually change for the stimuli\n%--------------------\n% Gabor information\n%--------------------\n% Obvious Parameters\norientation = 45;% in degrees, the angle of the lines.\naspectRatio = 1.0;\nphase = 0;\ndirection = 'R';\n% Change the temporal frequency of the drifting gradient\ndesiredfrequency = 4;\n% Spatial Frequency (Cycles Per Pixel)\n% One Cycle = Grey-Black-Grey-White-Grey i.e. One Black and One White Lobe\nnumCycles = 8;  % change the spatial frequency of the stimuli\n%contrasts = [1 .75 .5 .25  .125  .0625 .03125 .015625 .0078125 .00390625];\ncontrasts = [.75 .5 .25  .1875 .125 .09375 .0625 .03125 .015625 0];\n%contrasts = [ .175 .125 .09375 .0625 .05 .04 .03125 .023438 .015625 0];\n%contrasts = [   .125  .09375 .0625 0.055 .05 0.045 .04 .03125 .023438 .015625 0];\n%contrasts = [ 0.09  0.075 .06  0.055 .05 0.045 .04 0.035 .03 0.025  .02 .015  0.01 0];\n%contrasts = [ 0.1  0.0796 .0631  .0501 0.0398  0.0316 .0251 0.02  .0158 .0126  0.01 0];\n%contrasts = [ 0.09  0.075 .06  .05 0.04  0.035 .03 0.025  .02 .015  0.01 0];\n%contrasts = [.065 .06 .055 .05 .045 .04 .035 .03 .025 .02 .015 .01];\n%contrasts = [.045 .04 .035 .03 .025 .0225 .02 .0175 .015 .0125 .01 .005];  %M1\n%contrasts = [.045 .04 .035 .0325 .03 .0275 .025 .0225 .02 .0175 .015 .01]; % M2\n%contrasts = [.0228 .0201 .0156 .011 .0084];  %M1\n%contrasts = [0.0333 0.0314 0.0281 0.0248 0.023]; % M2\n%contrasts = [1  .5 .25  .125  .03125  .0078125 0];\n%contrasts = [1  .5 .25  .125  0];\ngo = 1;\nmaxc = round(numel(contrasts)/2);\n%%  To be run of not using exponential\n%%%%%%%%%%%%%%%%%%%%%%%%%%%%%%%%%%%%%%%%%%%%%%%%%%%%%%%%%%%%%%%%%%%%%%%%%%%%%%%%%%%%%%\n% This code will randomize the order of contrasts being presented\n[RandomizedTrials]=RandomizeTrials_Psuedo_function(contrasts,NT,'n');\n\n% This code will generate inter trial intervals with either random jitter\n% or based on an exponential distribution\nif goEXP < 1\n     jit = JIT;\n     jitter = rand(1,NT);\n     jitter = 2*jit*(jitter- .5);\n     ITIbase = BITI;\n     intervals = [ones(1,NT)*ITIbase];\n     intervals = intervals + jitter;\nelseif goEXP > 0\n     intervals = exponentialITI(1/lambda, minITI, maxITI, NT);\nend\n\n%%  Prep the stimulus presentation software\n%%%%%%%%%%%%%%%%%%%%%%%%%%%%%%%%%%%%%%%%%%%%%%%%%%%%%%%%%%%%%%%%%%%%%%%%%%%\n%Screen('Preference', 'SkipSyncTests', 1);\nsca;\nclose all;\n% Setup PTB with some default values\nPsychDefaultSetup(2);\n% Set the screen number to the external secondary monitor if there is one connected\nscreenNumber = max(Screen('Screens'));\n\n% Define black, white and grey\nwhite = WhiteIndex(screenNumber);\nblack = BlackIndex(screenNumber);\ngrey = white / 2;\n\n% Open the screen & define it's dimensions\n[window, windowRect] = PsychImaging('OpenWindow', screenNumber, grey,...\n    [], 32, 2, [], [], kPsychNeedRetinaResolution);\n[screenXpixels, screenYpixels] = Screen('WindowSize', window);\n[xCenter, yCenter] = RectCenter(windowRect);\n\n% Get the vertical refresh rate of the monitor\nifi = Screen('GetFlipInterval', window);\n\n% Set maximum priority level\ntopPriorityLevel = MaxPriority(window);\nPriority(topPriorityLevel);\n\n\n% Build a procedural gabor texture (Note: to get a \"standard\" Gabor patch\n% we set a grey background offset, disable normalisation, and set a\n% pre-contrast multiplier of 0.5).\n% Dimension of the region where will draw the Gabor in pixels\ngaborDimPix = windowRect(3);\n% Sigma of Gaussian  (how much to fade around the edges)\nsigma = gaborDimPix / 0;  % change the 0 value to alter the fading\nphasePerFrame = desiredfrequency*360*ifi;\nfreq = numCycles / gaborDimPix;\n\nbackgroundOffset = [0.5 0.5 0.5 0.0];\ndisableNorm = 1;\npreContrastMultiplier = 0.5;\ngabortex = CreateProceduralGabor(window, gaborDimPix, gaborDimPix, [],...\n    backgroundOffset, disableNorm, preContrastMultiplier);\n\n% Randomise the phase of the Gabors and make a properties matrix.\nfor N = 1:numel(contrasts)\npropertiesMat{1,N} = [phase, freq, sigma, contrasts(N), aspectRatio, 0, 0, 0];\nend\n\niiii = 1;\ncchoice = RandomizedTrials(iiii);\ncont2 = contrasts(cchoice);\npm = propertiesMat{1,1};\n\n\n%%  Build up the rectangles for the pause and hold screen\nbaseRect = [0 0 screenXpixels screenYpixels];\ncenteredRect = CenterRectOnPointd(baseRect, xCenter, yCenter);\nrectColorB = [0 0 0];\nrectColorG = [128 128 128]/255;\n\n%%  Finalize the trial data and orders\nstim_id = [ones(1,NT)*1];\nreward = [ones(1,NT)*1];\nmeanITI = nanmean(intervals);\nrand_idx1 = randperm(NT);\nrand_idx2 = randperm(NT);\nintervals = intervals(rand_idx2);\nstim_id = stim_id(rand_idx2);\nreward = reward(rand_idx2);\n%%  All Done!\n%  indicate that the necessary preloading of data has been completed.\nstim_loaded = 1;\n%%%\nconlim = .02;\nccc = sort(contrasts);\nif ccc(3) < conlim\n     conlim = ccc(3)\nend" ("Script Node")("NT"=w272, "BITI"=w271, "JIT"=w270, "cont"=w269, "goEXP"=w265, "minITI"=w264, "maxITI"=w263, "lambda"=w262) -> ("stim_loaded"=w277:dbl, "intervals"=w273:dbl[], "stim_id"=w274:dbl[], "reward"=w275:dbl[], "conlim"=w267:dbl, "meanITI"=→"meanITI":dbl)  [unwired: 1 in, 1 out]
            "stim_loaded" <- w277
            "Timings" <- w273
            "stim_id" <- w274
            "reward" <- w275
            n251 = shared-variable "My Computer\\michelle_library.lvlib\\Timings"(w273) -> ()  [unwired: 1 in, 1 out]
            n252 = shared-variable "My Computer\\michelle_library.lvlib\\Stim_ID"(w274) -> ()  [unwired: 1 in, 1 out]
            n253 = shared-variable "My Computer\\michelle_library.lvlib\\Reward_mat"(w275) -> ()  [unwired: 1 in, 1 out]
            n254 = shared-variable "My Computer\\michelle_library.lvlib\\EnticeLimiter"(w267) -> ()  [unwired: 1 in, 1 out]
            n255 = Equal?(x=w277, y=1.0) -> (x = y?=→"Stimuli Loaded?":bool)
          }
        }
        n256 = local read "Stimuli Loaded?"() -> (w258:bool)
      }
    }
    frame #3 {
      n257 = Get Date/Time In Seconds() -> (seconds since 1Jan1904=w284:timestamp)
      n258 = local read "Stimuli Loaded?"() -> (w279:bool)
      n259 = local read "Initialtime"() -> (w283:dbl)
      n260 = local read "Elapsed Time"() -> (w278:dbl)
      n261 = To Double Precision Float(number=w284) -> (double precision float=w281:dbl)
      n262 = shared-variable "My Computer\\michelle_library.lvlib\\InitiatedStamp"(w281) -> ()  [unwired: 1 in, 1 out]
      n263 = Subtract(x=w281, y=w283) -> (x-y=w282:dbl)
      n264 = shared-variable "My Computer\\michelle_library.lvlib\\Stim_loaded"(w279) -> ()  [unwired: 1 in, 1 out]
      n265 = Subtract(x=w278, y=w282) -> (x-y=→"Lag1":dbl)
      n266 = shared-variable "My Computer\\michelle_library.lvlib\\InitiatedLag"(w278) -> ()  [unwired: 1 in, 1 out]
    }
  }
